vi "Concurrent Access to TDMS File.vi"() -> ()   [LabVIEW 2023]
doc: "This example demonstrates concurrent access to the same TDMS file. Data is continuously appended to a TDMS file in one loop, while another loop reads from the file at the same time. As soon as data is added to the file, it will be available for reading. Move the scroll bar on the front panel to determine which portion of the file you want to display."
panel:
  out "Display start":u64
  in  "Stop":bool
  in  "Amplitude":dbl(slide)=51.57894736842105 scale=0.0..100.0
  in  "Frequency":dbl(slide)=50.526315789473685 scale=0.0..100.0
  out "Data written to file":waveform(dbl)(graph)
  out "Data read from file":waveform(dbl)(graph)
  in  "Scrollbar":u64(c297)
  out "Number of values in file":u64
  # "Overview: Demonstrates concurrent access to the same .tdms file. \nInstructions:\n1. Run the VI.\n2. Change the Frequency and Amplitude values to modify the generated data.\n3. Move the scroll bar under the Data read from file graph to specify which portion of the file you want to display.\n4. Click Stop to stop the VI.\n5. Delete the .tdms file (located at [LabVIEW Data]\\Example Concurrent Access.tdms) when you are done."
  # "Write Data to TDMS File"
  # "Read Data from TDMS File"
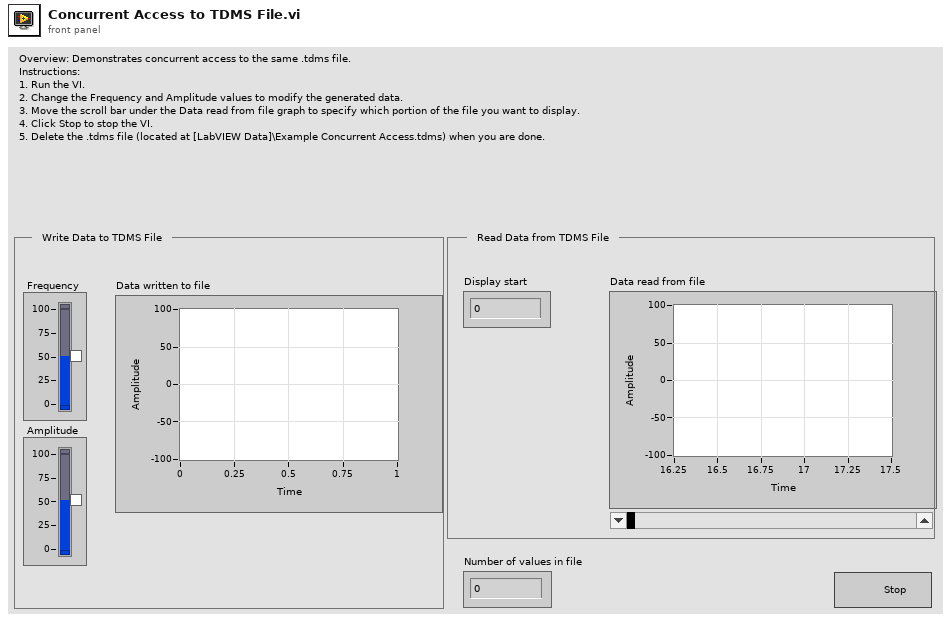
[diagram p1: front panel]
types:
  T1 = enum16{"open", "open or create", "create or replace", "create", "open (read-only)"}
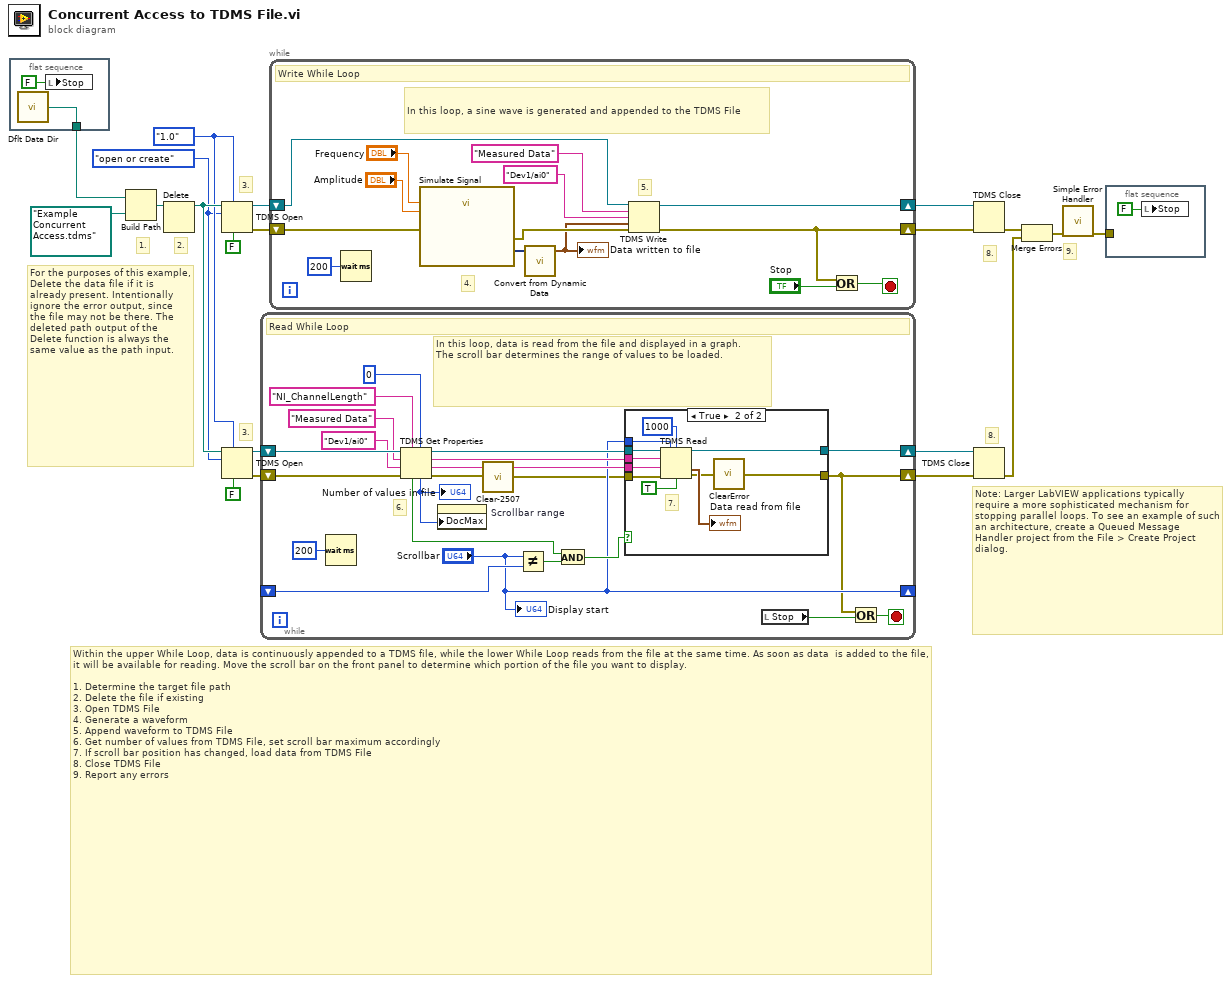
[diagram p0: block diagram]
diagram:
  w4 = enum16{"1.0", "2.0"}."1.0" ("file format version (2.0)")
  w3 = T1."open or create" ("operation")
  # "Note: Larger LabVIEW applications typically require a more sophisticated mechanism for stopping parallel loops. To see an example of such an architecture, create a Queued Message Handler project from the File > Create Project dialog."
  # "For the purposes of this example, Delete the data file if it is already present. Intentionally ignore the error output, since the file may not be there. The deleted path output of the Delete function is always the same value as the path input."
  # "9."
  # "8."
  # "8."
  # "3."
  # "3."
  # "2."
  # "1."
  # "Within the upper While Loop, data is continuously appended to a TDMS file, while the lower While Loop reads from the file at the same time. As soon as data  is added to the file, it will be available for reading. Move the scroll bar on the front panel to determine which portion of the file you want to display.\n\n1. Determine the target file path\n2. Delete the file if existing\n3. Open TDMS File\n4. Generate a waveform \n5. Append waveform to TDMS File\n6. Get number of values from TDMS File, set scroll bar maximum accordingly\n7. If scroll bar position has changed, load data from TDMS File\n8. Close TDMS File\n9. Report any errors"
  n1 = flat-sequence {
    tunnel: [w21] -> w2
    frame #0 {
      n2 = call <vilib>:"Dflt Data Dir.vi"() -> ("App:Default Data Directory"=w21:path)
      n3 = local write "Stop"(FALSE ("Stop")) -> ()
    }
  }
  n4 = Build Path(base path=w2, name or relative path=path "Example Concurrent Access.tdms" ("file path")) -> (appended path=w5:path)
  n5 = Delete(path (use dialog)=w5) -> (deleted path=w11:path)  [unwired: 1 in, 5 out]
  n6 = TDMS Open(6:FALSE ("disable buffering (T)"), 7:w4, 10:w3, 11:w11) -> (0:w15:errorcluster, 3:w14:refnum<k34>)  [unwired: 3 in]
  n7 = TDMS Open(6:FALSE ("disable buffering (T)"), 7:w4, 10:w3, 11:w11) -> (0:w18:errorcluster, 3:w19:refnum<k34>)  [unwired: 3 in]
  n8 = while {
    shift-right: [w25] -> w16
    shift-left: w18 -> [w43]
    shift-right: [w33] -> w17
    shift-left: w19 -> [w44]
    shift-right: ["Scrollbar"] -> _
    shift-left: _ -> [w36]
    stop <- w26 stop-if-true
    # "6."
    # "In this loop, data is read from the file and displayed in a graph. \nThe scroll bar determines the range of values to be loaded."
    # "Read While Loop"
    n9 = Wait (ms)(milliseconds to wait=u32 200) -> ()  [unwired: 1 out]
    n10 = TDMS Get Properties(5:u64 0, 7:"NI_ChannelLength" ("channel name(s) in"), 8:w43, 9:"Dev1/ai0" ("channel name"), 10:"Measured Data" ("channel name(s) in"), 11:w44) -> (0:w24:errorcluster, 1:w32:string, 2:w34:string, 3:w35:refnum<k34>, 4:w37:u64, 6:w30:bool)
    "Number of values in file" <- w37
    n11 = property on="Scrollbar range" class="Scroll (strict)"("DocMax"=w37) -> ()  [unwired: 2 in, 2 out]
    n12 = call <vilib>:"Clear-2507.vi"("error in (no error)"=w24) -> ("error out"=w23:errorcluster)
    n13 = Not Equal?(x="Scrollbar", y=w36) -> (x != y?=w31:bool)
    n14 = And(x=w30, y=w31) -> (x .and. y?=w29:bool)
    n15 = case shown="True" w29 {
      tunnel: w35 -> [w46 w57]
      tunnel: w23 -> [w45 w56]
      tunnel: w34 -> [_ w55]
      tunnel: [w45 w54] -> w25
      tunnel: [w46 w53] -> w33
      tunnel: w32 -> [_ w50]
      tunnel: "Scrollbar" -> [_ w47]
      frame False {
      }
      frame True {
        # "7."
        n16 = TDMS Read(0:w57, 1:w47, 2:i64 1000 ("count (-1: all)"), 5:w55, 7:w50, 11:w56, 13:TRUE ("return channels in file order? (F)")) -> (4:w53:refnum<k34>, 10:→"Data read from file":waveform(dbl), 15:w49:errorcluster)  [unwired: 1 in, 3 out]
        n17 = call <vilib>:"ClearError.vi"("error in (no error)"=w49) -> ("error out"=w54:errorcluster)
      }
    }
    n18 = local read "Stop"() -> (w27:bool)
    n19 = Or(x=w25, y=w27) -> (x .or. y?=w26:bool)
    "Display start" <- "Scrollbar"
  }
  n20 = while {
    shift-right: [w59] -> w13
    shift-left: w15 -> [w70]
    shift-right: [w69] -> w12
    shift-left: w14 -> [w71]
    stop <- w58 stop-if-true
    # "5."
    # "4."
    # "In this loop, a sine wave is generated and appended to the TDMS File"
    # "Write While Loop"
    n21 = Wait (ms)(milliseconds to wait=u32 200) -> ()  [unwired: 1 out]
    n22 = call "Simulate Signal"("Frequency"="Frequency", "Amplitude"="Amplitude", "error in (no error)"=w70) -> ("Sine"=w61:dynamicdata, "error out"=w67:errorcluster)  [unwired: 11 in]
    n23 = call "Convert from Dynamic Data"("Dynamic Data Type"=w61) -> ("Waveform"=w62:waveform(dbl))  [unwired: 3 in]
    "Data written to file" <- w62
    n24 = TDMS Write(0:w71, 5:"Measured Data" ("channel name(s) in"), 7:"Dev1/ai0" ("channel name"), 9:w62, 11:w67) -> (4:w69:refnum<k34>, 15:w59:errorcluster)  [unwired: 1 in, 2 out]
    n25 = Or(x=w59, y="Stop") -> (x .or. y?=w58:bool)
  }
  n26 = TDMS Close(8:w13, 11:w12) -> (0:w10:errorcluster)  [unwired: 1 out]
  n27 = TDMS Close(8:w16, 11:w17) -> (0:w9:errorcluster)  [unwired: 1 out]
  n28 = Merge Errors(w10, w9) -> (w8:errorcluster)
  n29 = call <vilib>:"Simple Error Handler.vi"("error in (no error)"=w8) -> ("error out"=w1:errorcluster)  [unwired: 1 in, 7 out]
  n30 = flat-sequence {
    tunnel: w1 -> [_]
    frame #0 {
      n31 = local write "Stop"(FALSE ("Stop")) -> ()
    }
  }
